vi "EJ 4.1.5 (final).vi"() -> ()   [LabVIEW 2013]
uses:
  <vilib>/gmath/statdist.llb/Normal Inverse CDF.vi
  <vilib>/gmath/NI_Gmath.lvlib
panel:
  in  "Vector":i64
  out "Waveform Chart":cluster{"x":dbl, dbl}(graph)
  in  "stop":bool
  in  "Nivel de ruido":dbl
  in  "Medicion":dbl
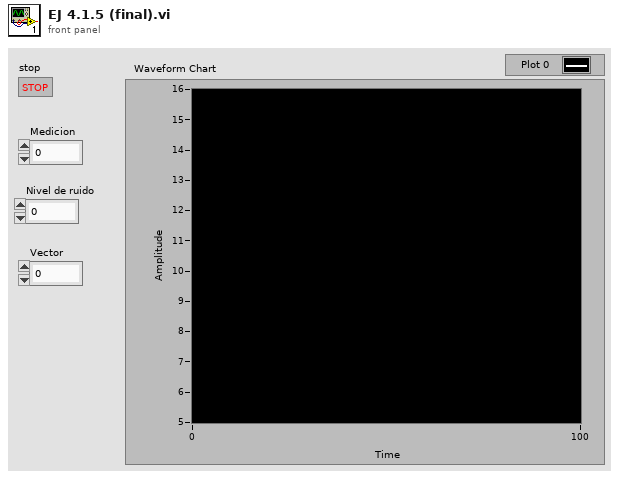
[diagram p1: front panel]
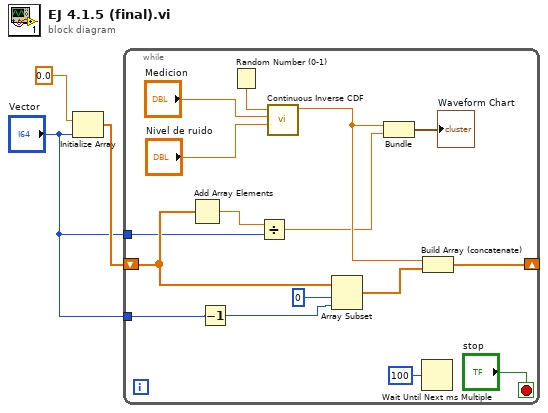
[diagram p0: block diagram]
diagram:
  n1 = Initialize Array(0.0, "Vector") -> (w2:dbl[])
  n2 = while {
    shift-right: [w13] -> _
    shift-left: w2 -> [w9]
    tunnel: "Vector" -> [w4]
    tunnel: "Vector" -> [w7]
    stop <- "stop" stop-if-true
    n3 = Add Array Elements(numeric array=w9) -> (sum=w8:dbl)
    n4 = Decrement(x=w4) -> (x-1=w5:i64)
    n5 = Random Number (0-1)() -> (number: 0 to 1=w15:dbl)
    n6 = Divide(x=w8, y=w7) -> (x/y=w6:dbl)
    n7 = call-poly <vilib>:"Continuous Inverse CDF.vi"("std"="Nivel de ruido", "mean"="Medicion", "cdf(x)"=w15) -> ("x"=w12:dbl)  [unwired: 7 in, 1 out]
    n8 = Array Subset(array=w9, index=0, length=w5) -> (w11:dbl[])
    n9 = Bundle("x"=w12, w6) -> (→"Waveform Chart":cluster{"x":dbl, dbl})  [unwired: 1 in]
    n10 = Wait Until Next ms Multiple(millisecond multiple=u32 100) -> ()  [unwired: 1 out]
    n11 = Build Array (concatenate)(w12, w11) -> (w13:dbl[])
  }
